vi "Get File Size.vi"(8 "error in (no error)":errorcluster, 10 "Remote FileName":string, 11 "FTP in":refnum<class "FTP.lvclass">) -> (0 "error out":errorcluster, 2 "FileSize":i64, 3 "FTP out":refnum<class "FTP.lvclass">)   [LabVIEW 2017, in "FTP_UpgradeCSMF.lvlib" / "FTP.lvclass"]
doc: "This vi will return the size of the file specified by the \"Remote FileName\" parameter. Not all FTP servers will respond to this command. Only servers that have the SIZE feature will respond appropriately."
uses:
  FTP.lvclass
  FTP.lvclass/FTP.ctl
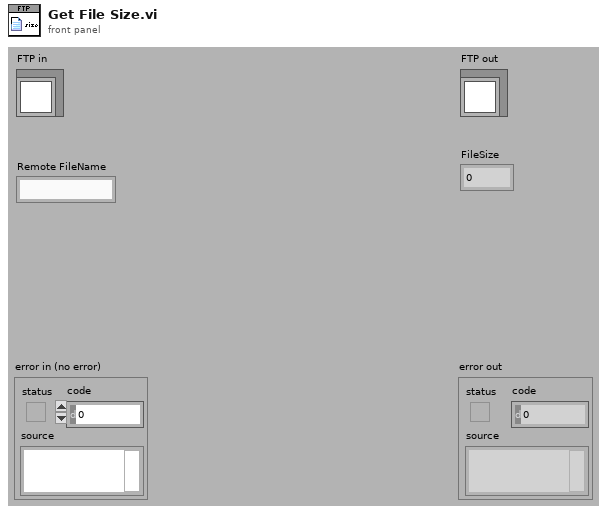
[diagram p1: front panel]
types:
  T1 = typedef "FTP_UpgradeCSMF.lvlib/FTP.lvclass/Dir-File Info.ctl" = cluster{"Name":string, "Modify Timestamp":timestamp, "Dir-File Type":T2, "Unique Id":string, "Permissions":string, "Unix Mode":u16, "Owner":string, "Group":string, "FileSize":i64}
  T2 = typedef "FTP_UpgradeCSMF.lvlib/FTP.lvclass/Dir-File Type.ctl" = enum16{"File", "Listed Directory", "Parent Directory", "Directory", "Unknown"}
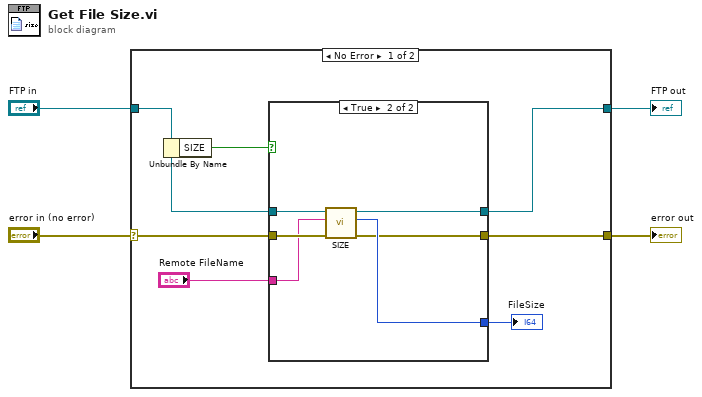
[diagram p0: block diagram]
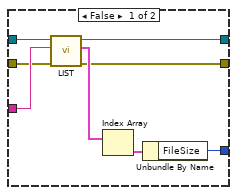
[diagram p2: hidden frame]
diagram:
  n1 = case shown="No Error" "error in (no error)" {
    selector: "error in (no error)" -> [w6 w27]
    tunnel: [w11 w27] -> w3
    tunnel: [w10 w26] -> w1
    tunnel: "FTP in" -> [w5 w26]
    frame No Error {
      n2 = Unbundle By Name(w5) -> ("SIZE"=w7:bool)
      n3 = case shown="True" w7 {
        tunnel: [w13 w23] -> w11
        tunnel: w5 -> [w19 w21]
        tunnel: [w18 w20] -> w10
        tunnel: "Remote FileName" -> [w17 w22]
        tunnel: [w14 w24] -> w8
        tunnel: w6 -> [w12 w25]
        frame False {
          n4 = call "LIST.vi"("error in (no error)"=w12, "Remote File"=w17, "FTP in"=w19) -> ("error out"=w13:errorcluster, "Dir-File Info Array"=w16:T1[], "FTP out"=w18:refnum<class "FTP.lvclass">)  [unwired: 6 in]
          n5 = Index Array(array=w16) -> (element=w15:T1)  [unwired: 1 in]
          n6 = Unbundle By Name(w15) -> ("FileSize"=w14:i64)
        }
        frame True {
          n7 = call "SIZE.vi"("error in (no error)"=w25, "Remote FileName"=w22, "FTP in"=w21) -> ("error out"=w23:errorcluster, "FileSize"=w24:i64, "FTP out"=w20:refnum<class "FTP.lvclass">)  [unwired: 6 in]
        }
      }
      "FileSize" <- w8
    }
    frame Error {
    }
  }
  "error out" <- w3
  "FTP out" <- w1
